vi "perform.vi"(8 "error in (no error)":errorcluster, 11 "MissionQueue in":refnum<class "MissionQueue.lvclass">) -> (0 "error out":errorcluster, 1 "Valid?":bool, 2 "Desired Location":T1 {"North" format="%#_10f"; "East" format="%#_8f"}, 3 "MissionQueue out":refnum<class "MissionQueue.lvclass">)   [LabVIEW 2011, in "MissionQueue.lvclass"]
uses:
  MissionQueue.lvclass
  2 Typedefs/UTM Location.ctl
  Missions/GenericMission/GenericMission.lvclass
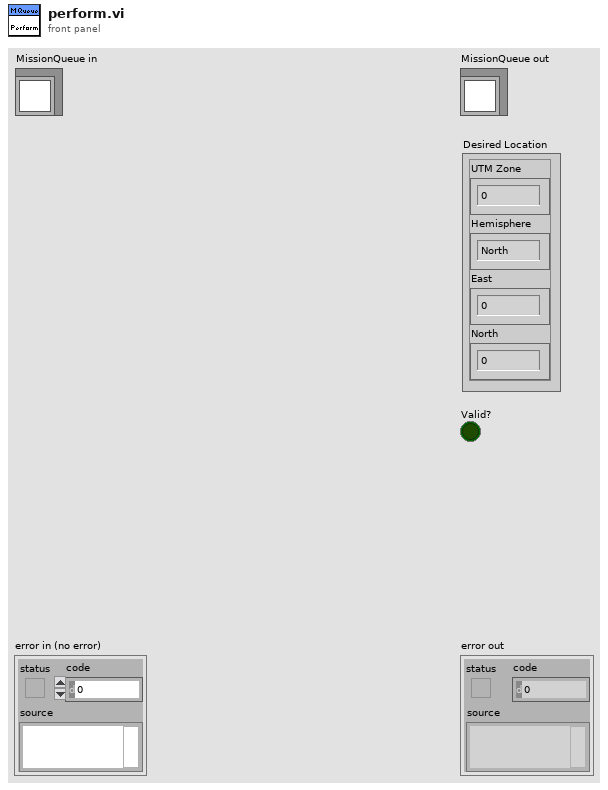
[diagram p1: front panel]
types:
  T1 = typedef "UTM Location.ctl" = cluster{"UTM Zone":i32, "Hemisphere":enum16{"North", "South"}, "East":dbl, "North":dbl}
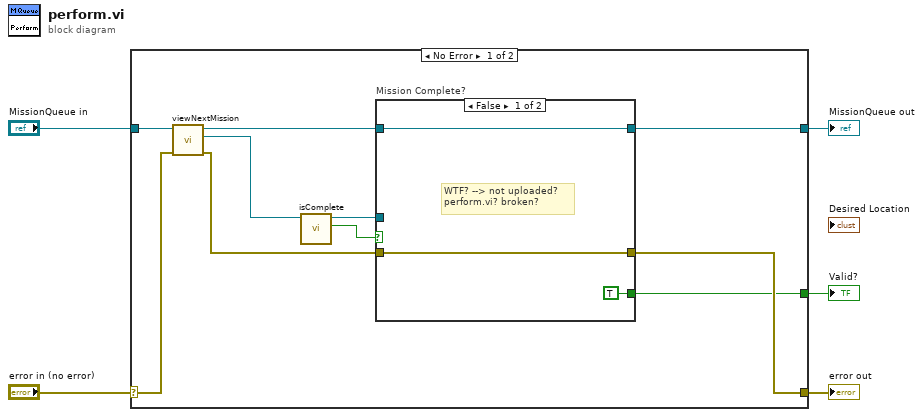
[diagram p0: block diagram]
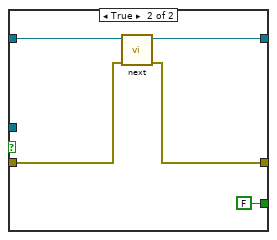
[diagram p2: hidden frame]
diagram:
  n1 = case shown="No Error" "error in (no error)" {
    selector: "error in (no error)" -> [w10 w25]
    tunnel: [w15 w25] -> w4
    tunnel: [w14 w24] -> w2
    tunnel: "MissionQueue in" -> [w12 w24]
    tunnel: [w13 _] -> w1
    frame No Error {
      n2 = call "viewNextMission.vi"("error in (no error)"=w10, "MissionQueue in"=w12) -> ("error out"=w6:errorcluster, "GenericMission.lvclass"=w9:refnum<class "GenericMission.lvclass">, "MissionQueue out"=w11:refnum<class "MissionQueue.lvclass">)  [unwired: 6 in, 1 out]
      n3 = call-dynamic "isComplete.vi"("Mission in"=w9) -> ("Mission Complete?"=w7:bool, "Mission out"=w8:refnum<class "GenericMission.lvclass">)  [unwired: 8 in, 1 out]
      n4 = case "Mission Complete?" shown="False" w7 {
        tunnel: w8 -> [_ _]
        tunnel: w6 -> [w16 w21]
        tunnel: [w16 w20] -> w15
        tunnel: w11 -> [w18 w23]
        tunnel: [w18 w22] -> w14
        tunnel: [TRUE ("Valid?") FALSE ("Valid?")] -> w13
        frame False {
          # "WTF? --> not uploaded?\nperform.vi? broken?"
        }
        frame True {
          n5 = call "next.vi"("error in (no error)"=w21, "MissionQueue in"=w23) -> ("error out"=w20:errorcluster, "MissionQueue out"=w22:refnum<class "MissionQueue.lvclass">)  [unwired: 6 in, 2 out]
        }
      }
    }
    frame Error {
    }
  }
  "error out" <- w4
  "MissionQueue out" <- w2
  "Valid?" <- w1
